vi "Send Event.vi"(7 "Priority Message":bool, 8 "error in":errorcluster, 9 "Payload":variant, 10 "Command":string) -> (0 "error out":errorcluster)   [LabVIEW 2020, in "GUI.lvlib"]
uses:
  GUI.lvlib
  Eventing/Event Type.ctl
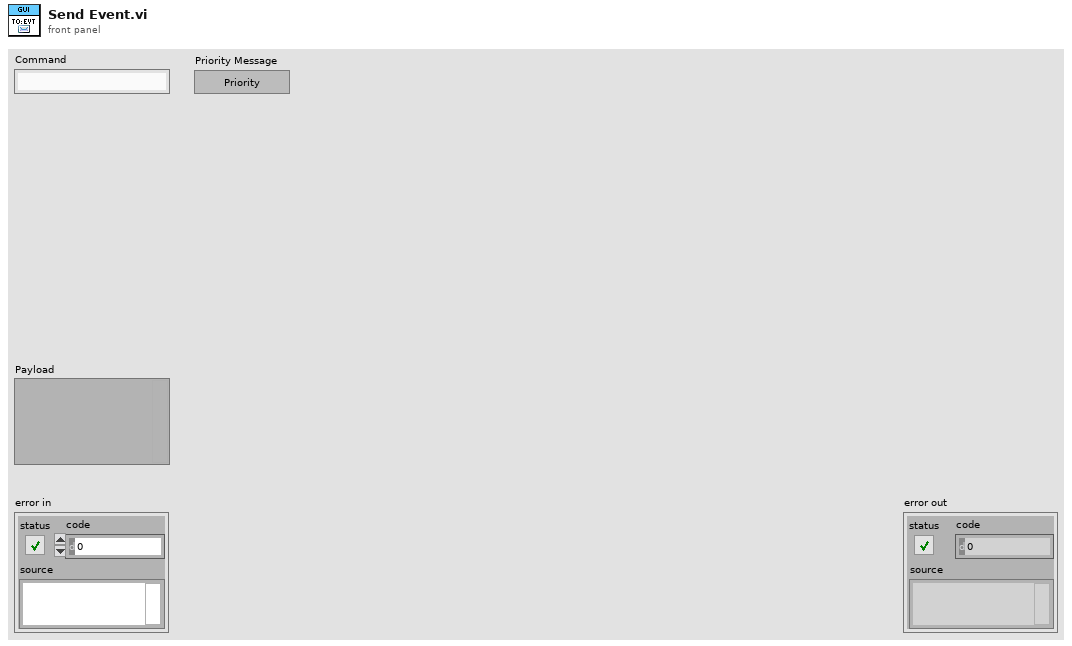
[diagram p1: front panel]
types:
  T1 = typedef "GUI.lvlib/Event Type.ctl" = cluster{"Command":string, "Payload":variant}
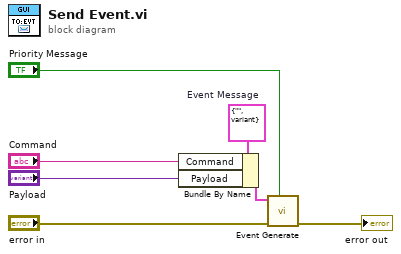
[diagram p0: block diagram]
diagram:
  w7 = T1 {"Command"="", "Payload"=variant}  # Event Message
  n1 = Bundle By Name(cluster=w7, "Command"="Command", "Payload"="Payload") -> (w5:T1)
  n2 = call "Event Generate.vi"("Priority Message"="Priority Message", "error in"="error in", "Event Type"=w5) -> ("error out"=→"error out":errorcluster)  [unwired: 8 in]
